vi "SaveConfiguration.vi"(11 "Handle":u32) -> (3 "FT_Status":u32(ring) items=["FT_OK", "FT_INVALID_HANDLE", "FT_DEVICE_NOT_FOUND", "FT_DEVICE_NOT_OPENED", "FT_IO_ERROR", "FT_INSUFFICIENT_RESOURCES", "FT_INVALID_PARAMETER", "FT_INVALID_BAUD_RATE", "FT_DEVICE_NOT_OPENED_FOR_ERASE", "FT_DEVICE_NOT_OPENED_FOR_WRITE", "FT_FAILED_TO_WRITE_DEVICE", "FT_EEPROM_READ_FAILED", "FT_EEPROM_WRITE_FAILED", "FT_EEPROM_ERASE_FAILED", "FT_EEPROM_NOT_PRESENT", "FT_EEPROM_NOT_PROGRAMMED", "FT_INVALID_ARGS", "FT_NOT_SUPPORTED", "FT_OTHER_ERROR"])   [LabVIEW 2011]
panel:
  out "SaveStatus":i32
  out "Bytes Written":u32
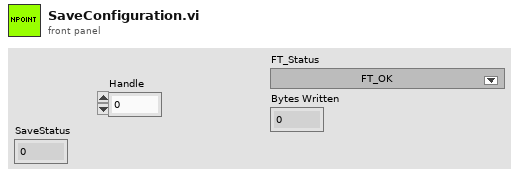
[diagram p1: front panel]
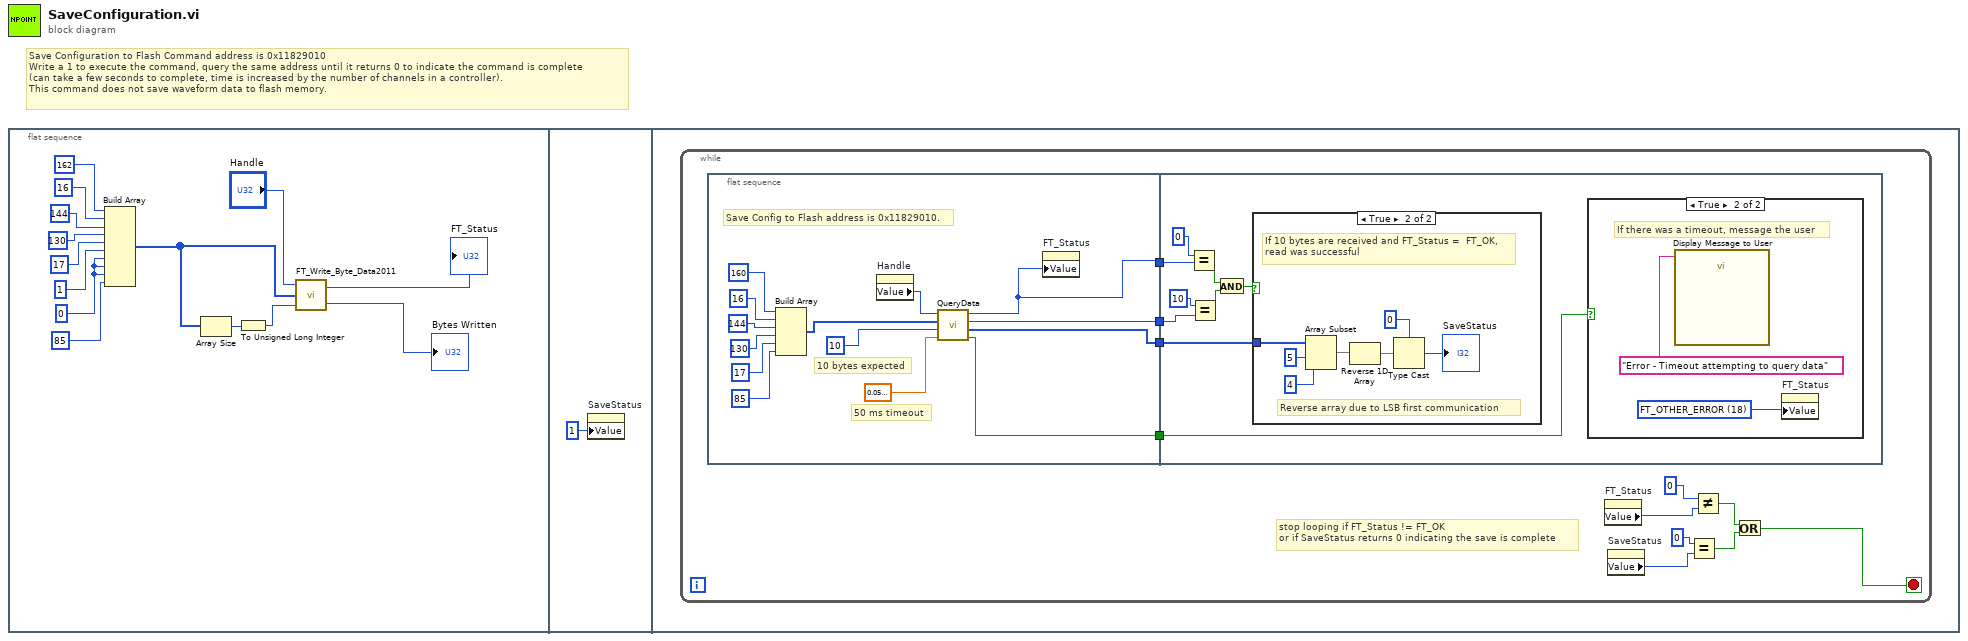
[diagram p0: block diagram]
diagram:
  # "Save Configuration to Flash Command address is 0x11829010\nWrite a 1 to execute the command, query the same address until it returns 0 to indicate the command is complete\n(can take a few seconds to complete, time is increased by the number of channels in a controller).\nThis command does not save waveform data to flash memory."
  n1 = flat-sequence {
    frame #0 {
      w2 = u8 0 ("element")
      n2 = Build Array(u8 162 ("element"), u8 16 ("element"), u8 144 ("element"), u8 130 ("element"), u8 17 ("element"), u8 1 ("element"), w2, w2, w2, u8 85 ("element")) -> (w6:u8[])
      n3 = Array Size(array=w6) -> (size(s)=w14:i32)
      n4 = To Unsigned Long Integer(number=w14) -> (unsigned 32bit integer=w13:u32)
      n5 = call "FT_Write_Byte_Data2011.vi"("Bytes To Write"=w13, "Buffer"=w6, "Handle"="Handle") -> ("Bytes Written"=→"Bytes Written":u32, "FT_Status"=→"FT_Status":u32)
    }
    frame #1 {
      n6 = property on="SaveStatus" class="DigNum (strict)"("Value"=1 ("SaveStatus")) -> ()  [unwired: 2 in, 2 out]
    }
    frame #2 {
      n7 = while {
        stop <- w19 stop-if-true
        # "stop looping if FT_Status != FT_OK\nor if SaveStatus returns 0 indicating the save is complete"
        n8 = flat-sequence {
          tunnel: [w32] -> w26
          tunnel: [w31] -> w25
          tunnel: [w30] -> w24
          tunnel: [w28] -> w23
          tunnel: w26 -> [w49]
          tunnel: w25 -> [w47]
          tunnel: w24 -> [w46]
          tunnel: w23 -> [w44]
          frame #0 {
            # "10 bytes expected"
            # "50 ms timeout"
            # "Save Config to Flash address is 0x11829010."
            n9 = Build Array(u8 160 ("element"), u8 16 ("element"), u8 144 ("element"), u8 130 ("element"), u8 17 ("element"), u8 85 ("element")) -> (w35:u8[])
            n10 = property on="Handle" class="DigNum (strict)"() -> ("Value"=w27:u32)  [unwired: 2 in, 2 out]
            n11 = call "QueryData.vi"("TimeoutLengthSeconds"=sgl 0.05, "NumBytesExpected"=u32 10, "Message"=w35, "Handle"=w27) -> ("Timeout"=w30:bool, "Return Array"=w31:u8[], "Bytes Read"=w32:u32, "FT_Status"=w28:u32)  [unwired: 4 in]
            n12 = property on="FT_Status" class="Ring (strict)"("Value"=w28) -> ()  [unwired: 2 in, 2 out]
          }
          frame #1 {
            n13 = Equal?(x=u32 0, y=w44) -> (x = y?=w42:bool)
            n14 = Equal?(x=u32 10, y=w49) -> (x = y?=w43:bool)
            n15 = And(x=w42, y=w43) -> (x .and. y?=w41:bool)
            n16 = case shown="True" w41 {
              tunnel: w47 -> [_ w58]
              frame False {
              }
              frame True {
                # "Reverse array due to LSB first communication"
                # "If 10 bytes are received and FT_Status =  FT_OK,\nread was successful"
                n17 = Array Subset(array=w58, index=5, length=4) -> (w54:u8[])
                n18 = Reverse 1D Array(array=w54) -> (reversed array=w53:u8[])
                n19 = Type Cast(type=0, x=w53) -> (*(type *) &x=→"SaveStatus":i32)
              }
            }
            n20 = case shown="True" w46 {
              frame False {
              }
              frame True {
                w50 = u32 18 items=["FT_OK", "FT_INVALID_HANDLE", "FT_DEVICE_NOT_FOUND", "FT_DEVICE_NOT_OPENED", "FT_IO_ERROR", "FT_INSUFFICIENT_RESOURCES", "FT_INVALID_PARAMETER", "FT_INVALID_BAUD_RATE", "FT_DEVICE_NOT_OPENED_FOR_ERASE", "FT_DEVICE_NOT_OPENED_FOR_WRITE", "FT_FAILED_TO_WRITE_DEVICE", "FT_EEPROM_READ_FAILED", "FT_EEPROM_WRITE_FAILED", "FT_EEPROM_ERASE_FAILED", "FT_EEPROM_NOT_PRESENT", "FT_EEPROM_NOT_PROGRAMMED", "FT_INVALID_ARGS", "FT_NOT_SUPPORTED", "FT_OTHER_ERROR"] ("FT_Status")
                # "If there was a timeout, message the user"
                n21 = call "Display Message to User"("Message"="Error - Timeout attempting to query data") -> ()  [unwired: 9 in, 2 out]
                n22 = property on="FT_Status" class="Ring (strict)"("Value"=w50) -> ()  [unwired: 2 in, 2 out]
              }
            }
          }
        }
        n23 = property on="FT_Status" class="Ring (strict)"() -> ("Value"=w21:u32)  [unwired: 2 in, 2 out]
        n24 = property on="SaveStatus" class="DigNum (strict)"() -> ("Value"=w17:i32)  [unwired: 2 in, 2 out]
        n25 = Equal?(x=u32 0, y=w17) -> (x = y?=w16:bool)
        n26 = Not Equal?(x=u32 0, y=w21) -> (x != y?=w20:bool)
        n27 = Or(x=w20, y=w16) -> (x .or. y?=w19:bool)
      }
    }
  }
